vi "AssertSubpanelVIName_Tests.vi"(11 "error in":errorcluster) -> (15 "error out":errorcluster)   [LabVIEW 2016, in "DronaTest.lvlib"]
uses:
  DronaTest.lvlib
  APIs/Stimulus/ControlValue/SetValueAuto.vi
  APIs/Assert/AssertControlValue/Controls/Subpanel/AssertSubpanelVI.vi
  <vilib>/addons/_JKI Toolkits/Caraya/classes/Assert/Assert Error.vi
  <vilib>/addons/_JKI Toolkits/Caraya/classes/Assert/Assert Equal Value_Variant.vi
  APIs/Assert/AssertControlValue/Controls/Subpanel/AssertSubpanel.lvlib
  <vilib>/addons/_JKI Toolkits/Caraya/classes/Assert/Assert.lvclass
  Drona.lvlib
  <vilib>/addons/_JKI Toolkits/Caraya/classes/Test/Test.lvclass
  APIs/Stimulus/ControlValue/ControlValue.lvlib
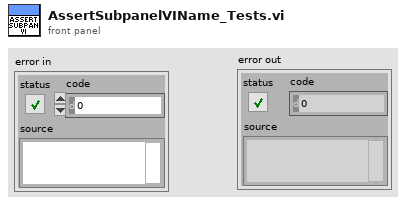
[diagram p1: front panel]
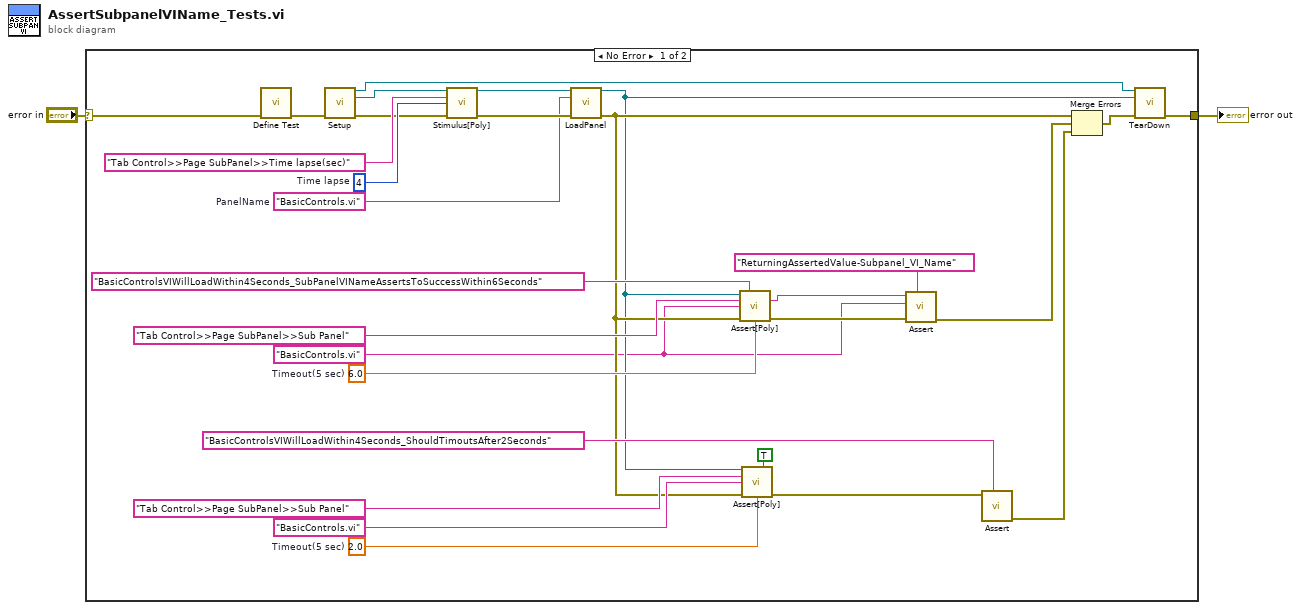
[diagram p0: block diagram]
diagram:
  n1 = case shown="No Error" "error in" {
    selector: "error in" -> [w28 w32]
    tunnel: [w13 w32] -> w1
    frame No Error {
      w25 = "BasicControls.vi"  # PanelName
      w29 = u32 4  # Time lapse
      w21 = 2.0  # Timeout(5 sec)
      w16 = 6.0  # Timeout(5 sec)
      w4 = "BasicControls.vi" ("VI Name")
      n2 = call <vilib>:"Define Test.vi"("error in (no error)"=w28) -> ("error out"=w15:errorcluster)  [unwired: 9 in, 1 out]
      n3 = call "Setup.vi"("error in"=w15) -> ("Application Ref"=w12:refnum<vi>, "VI out"=w9:refnum<vi>, "error out"=w11:errorcluster)  [unwired: 12 in]
      n4 = call-poly "Stimulus[Poly].vi"("VI Reference In"=w9, "Control Path"="Tab Control>>Page SubPanel>>Time lapse(sec)", "Value (Signaling)"=w29, "error in"=w11) -> ("VI Reference Out"=w27:refnum<vi>, "error out"=w26:errorcluster)  [unwired: 10 in]
      n5 = call "LoadPanel.vi"("VI in"=w27, "Item Name"=w25, "error in"=w26) -> ("VI out"=w8:refnum<vi>, "error out"=w10:errorcluster)  [unwired: 11 in]
      n6 = call-poly "Assert[Poly].vi"("VI Reference In"=w8, "Test Label"="BasicControlsVIWillLoadWithin4Seconds_SubPanelVINameAssertsToSuccessWithin6Seconds" ("Label"), "Control Path"="Tab Control>>Page SubPanel>>Sub Panel", "VI Name"=w4, "Error In"=w10, "Timeout(5 sec)"=w16) -> ("Asserted Value"=w5:string, "Error Out"=w7:errorcluster)  [unwired: 7 in, 1 out]
      n7 = call-poly "Assert[Poly].vi"("VI Reference In"=w8, "Assert Only? (F)"=TRUE, "Control Path"="Tab Control>>Page SubPanel>>Sub Panel", "VI Name"="BasicControls.vi", "Error In"=w10, "Timeout(5 sec)"=w21) -> ("Error Out"=w19:errorcluster)  [unwired: 7 in, 2 out]
      n8 = call-poly <vilib>:"Assert.vi"("Label"="ReturningAssertedValue-Subpanel_VI_Name", "error in (no error)"=w7, "Y"=w4, "X"=w5) -> ("error out"=w6:errorcluster)  [unwired: 6 in, 1 out]
      n9 = call-poly <vilib>:"Assert.vi"("Label"="BasicControlsVIWillLoadWithin4Seconds_ShouldTimoutsAfter2Seconds", "Error?"=w19) -> ("error out"=w31:errorcluster)  [unwired: 8 in, 1 out]
      n10 = Merge Errors(w10, w6, w31) -> (w14:errorcluster)
      n11 = call "TearDown.vi"("Application Ref"=w12, "VI in"=w8, "error in (no error)"=w14) -> ("error out"=w13:errorcluster)  [unwired: 12 in]
    }
    frame Error {
    }
  }
  "error out" <- w1
